vi "Ultramat 23 Initialize.vi"(0 "VISA resource name":refnum<visa-resource-name>="OXYMAT", 5 "Source Address":u8=208 format="%.0x", 7 "Target Address":u8=16 format="%.0x", 11 "error in (no error)":errorcluster) -> (4 "VISA Session Out":refnum<visa-resource-name>, 6 "Message Header":T1 {"Source Address" format="%.0x"; "Target Address" format="%.0x"}, 8 "Channel Type":T3(ring), 10 "Channel":T4, 14 "Success":bool, 15 "error out":errorcluster)   [LabVIEW 2023]
uses:
  instr.lib/Siemens ELAN/Message Header.ctl
  instr.lib/Siemens ELAN/Channel Status.ctl
  instr.lib/Siemens ELAN/Siemens ELAN.lvlib
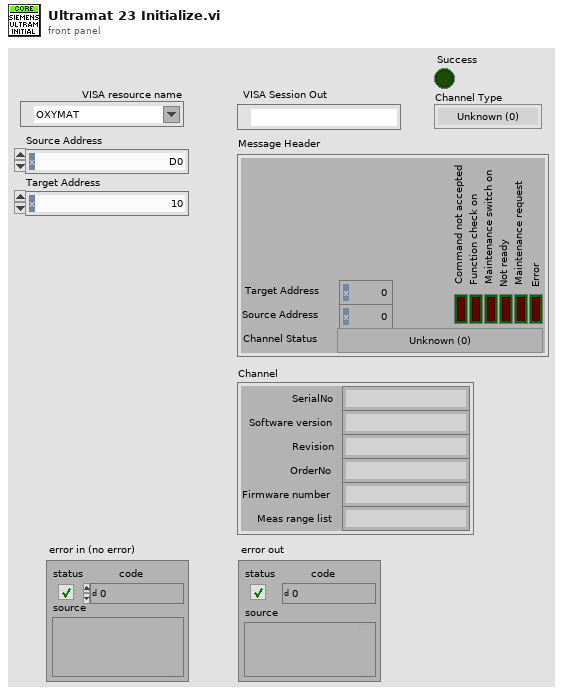
[diagram p1: front panel]
types:
  T1 = typedef "Siemens ELAN.lvlib/Message Header.ctl" = cluster{"Target Address":u8, "Source Address":u8, "Error":bool, "Maintenance request":bool, "Not ready":bool, "Maintenance switch on":bool, "Function check on":bool, "Command not accepted":bool, "Channel Status":T2}
  T2 = typedef "Siemens ELAN.lvlib/Channel Status.ctl" = enum8{"Unknown (0)", "Warm-up", "Pause", "Standby", "Measure", "Zero calibration", "Adjust component slope", "Unknown (7)", "Adjust curve dip", "Adjust linearization sensitivity", "Adjust temperature compensation", "Adjust pressure compensation", "Adjust linearization zero", "Adjust flow sensor", "Autocal", "Adjust phase", "Zero calibration of O2 sensor", "Synchronous zero calibration", "Purging for synchronous zero calibration", "Adjust analog output", "Adjust analog input", "Cleaning", "Unknown (>21)"}
  T3 = enum8{"Unknown (0)", "ULTRAMAT 6", "OXYMAT 6", "FIDAMAT 6", "ULTRAMAT 23", "SIPAN 34", "Unknown (6)", "CALOMAT 6", "Unknown (>7)"}
  T4 = cluster{"SerialNo":string, "Software version":string, "Revision":string, "OrderNo":string, "Firmware number":string, "Meas range list":string}
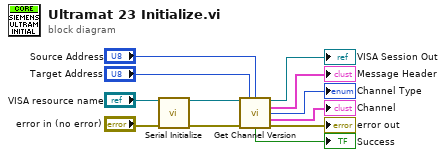
[diagram p0: block diagram]
diagram:
  n1 = call "Serial Initialize.vi"("VISA Session In"="VISA resource name", "error in (no error)"="error in (no error)") -> ("VISA Session Out"=w8:refnum<visa-resource-name>, "error out"=w9:errorcluster)  [unwired: 12 in]
  n2 = call "Get Channel Version.vi"("VISA Session In"=w8, "Target Address"="Target Address", "Source Address"="Source Address", "error in (no error)"=w9) -> ("VISA Session Out"=→"VISA Session Out":refnum<visa-resource-name>, "Message Header"=→"Message Header":T1, "Channel Type"=→"Channel Type":T3, "Channel"=→"Channel":T4, "Success"=→"Success":bool, "error out"=→"error out":errorcluster)  [unwired: 6 in]
